vi "Untitled 1.vi"   [LabVIEW 2015]
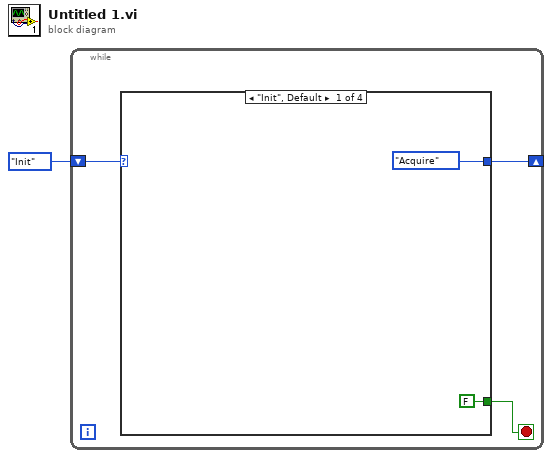
[diagram p0: block diagram]
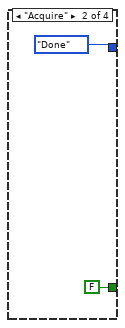
[diagram p2: hidden frame]
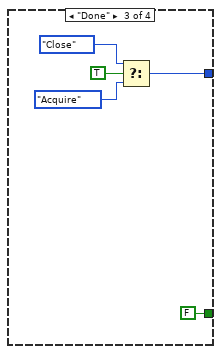
[diagram p3: hidden frame]
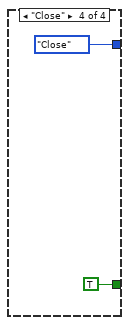
[diagram p4: hidden frame]
diagram:
  n1 = while {
    shift-right: [w3] -> _
    shift-left: enum16{"Init", "Acquire", "Done", "Close"}."Init" -> [w4]
    stop <- w2 stop-if-true
    n2 = case shown="\"Init\", Default" w4 {
      tunnel: [enum16{"Init", "Acquire", "Done", "Close"}."Acquire" enum16{"Init", "Acquire", "Done", "Close"}."Done" w10 enum16{"Init", "Acquire", "Done", "Close"}."Close"] -> w3
      tunnel: [FALSE FALSE FALSE TRUE] -> w2
      frame "Init", Default {
      }
      frame "Acquire" {
      }
      frame "Done" {
        n3 = Select(t=enum16{"Init", "Acquire", "Done", "Close"}."Close", s=TRUE, f=enum16{"Init", "Acquire", "Done", "Close"}."Acquire") -> (s? t:f=w10:enum16{"Init", "Acquire", "Done", "Close"})
      }
      frame "Close" {
      }
    }
  }
